vi "PublishCurrentValues.vi"(8 "error in (no error)":errorcluster, 10 "Qbus in":refnum<class "Qbus.lvclass">, 11 "config in":T1) -> (0 "error out":errorcluster, 3 "config out":T1)   [LabVIEW 2017, in "TestPanel.lvlib"]
uses:
  <vilib>/addons/InsightCM/Devices/Shared/Common/TestPanel/TestPanel.lvlib
  <vilib>/addons/InsightCM/Devices/Shared/Common/TestPanel/controls/Configuration.ctl
  <vilib>/addons/InsightCM/Devices/Shared/Common/TestPanel/controls/State.ctl
  <vilib>/addons/InsightCM/MessageBus/Base/controls/IRoutingSource.ctl
  <vilib>/addons/Qbus/Qbus.lvclass
  <vilib>/addons/InsightCM/MessageBus/MessageLibrary/Device/controls/DeviceTestPanelGetCurrentValuesResponseBody.ctl
  <vilib>/addons/InsightCM/MessageBus/Base/controls/TestPanelCurrentValues.ctl
  <vilib>/addons/InsightCM/MessageBus/Base/controls/KeyValuePair.ctl
  <vilib>/addons/InsightCM/MessageBus/Base/controls/TestPanelCurrentValue.ctl
  <vilib>/addons/InsightCM/MessageBus/Base/controls/TestPanelValue.ctl
  <vilib>/addons/InsightCM/Devices/Shared/Common/ServerComm/ServerComm.lvlib
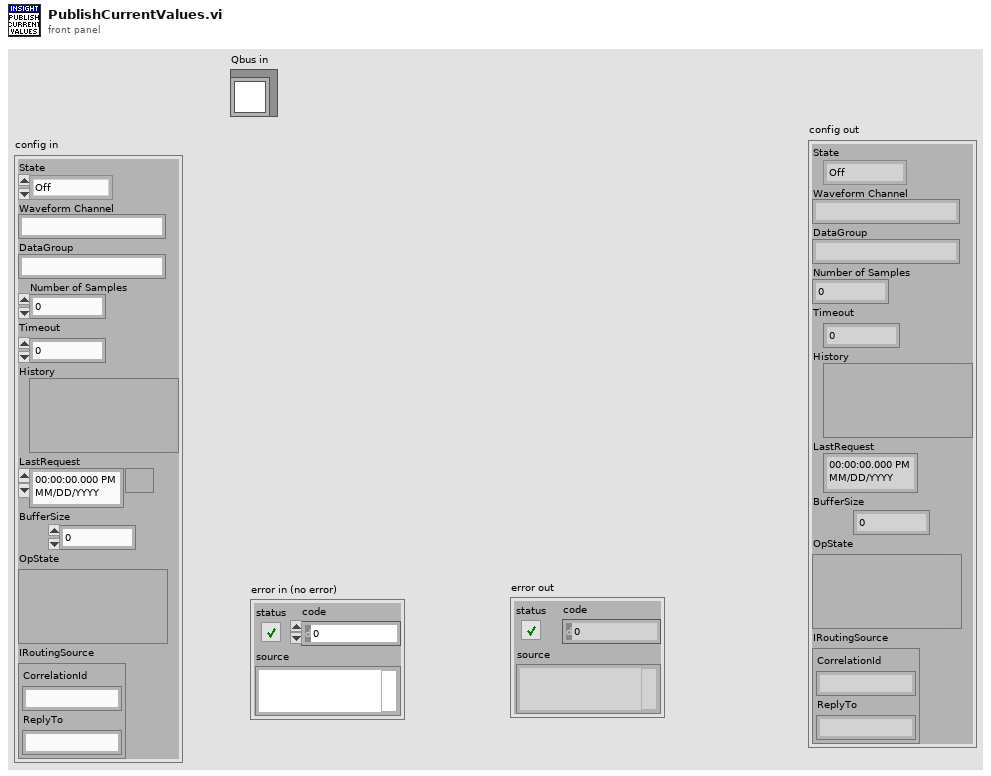
[diagram p1: front panel]
types:
  T1 = typedef "TestPanel.lvlib/Configuration.ctl" = cluster{"State":T2, "Waveform Channel":string, "DataGroup":string, "Number of Samples":i32, "Timeout":dbl, "History":variant, "LastRequest":timestamp, "BufferSize":i32, "OpState":variant, "IRoutingSource":T3}
  T2 = typedef "TestPanel.lvlib/State.ctl" = enum16{"Off", "On", "PendingValues", "PendingDataSet"}
  T3 = typedef "IRoutingSource.ctl" = cluster{"CorrelationId":string, "ReplyTo":string}
  T4 = typedef "DeviceTestPanelGetCurrentValuesResponseBody.ctl" = cluster{"Data":T5[]}
  T5 = typedef "TestPanelCurrentValues.ctl" = cluster{"DataGroup":string, "OperatingState":string, "ChannelStatus":T6[], "Values":T7[]}
  T6 = typedef "KeyValuePair.ctl" = cluster{"Key":string, "Value":string}
  T7 = typedef "TestPanelCurrentValue.ctl" = cluster{"TrendPointId":string, "AssetName":string, "MetricName":string, "Unit":string, "Value":T8}
  T8 = typedef "TestPanelValue.ctl" = cluster{"Value":dbl, "Timestamp":i64, "Invalid":bool}
  T9 = typedef "Message.ctl" = cluster{"Header":T10, "Body":u8[]}
  T10 = typedef "MessageHeader.ctl" = cluster{"MessageName":string, "Timestamp":i64, "CorrelationId":string, "ContentType":string, "RoutingKey":string, "Properties":T6[]}
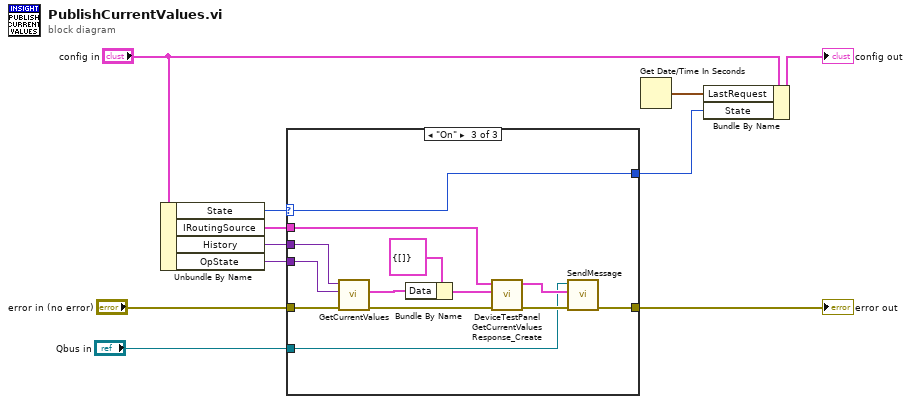
[diagram p0: block diagram]
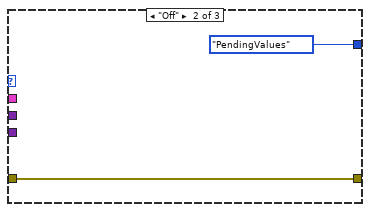
[diagram p3: hidden frame]
diagram:
  n1 = Unbundle By Name("config in") -> ("State"=w8:T2, "IRoutingSource"=w4:T3, "History"=w7:variant, "OpState"=w6:variant)
  n2 = case shown="\"On\"" w8 {
    selector: w8 -> [w13 _ w16]
    tunnel: w7 -> [_ _ w28]
    tunnel: w6 -> [_ _ w27]
    tunnel: "error in (no error)" -> [w12 w14 w23]
    tunnel: w4 -> [_ _ w21]
    tunnel: "Qbus in" -> [_ _ w18]
    tunnel: [w12 w14 w17] -> w2
    tunnel: [w13 State."PendingValues" ("State") w16] -> w1
    frame Default {
    }
    frame "Off" {
    }
    frame "On" {
      n3 = call <vilib>:"GetCurrentValues.vi"("error in (no error)"=w23, "OpState"=w27, "History"=w28) -> ("error out"=w22:errorcluster, "current values"=w25:T5[])  [unwired: 7 in]
      n4 = Bundle By Name(cluster=T4 {"Data"=[]} ("DeviceTestPanelGetCurrentValuesResponse"), "Data"=w25) -> (w24:T4)
      n5 = call <vilib>:"DeviceTestPanelGetCurrentValuesResponse_Create.vi"("error in (no error)"=w22, "DeviceTestPanelGetCurrentValuesResponse"=w24, "IRoutingSource"=w21) -> ("error out"=w20:errorcluster, "Message"=w19:T9)  [unwired: 7 in]
      n6 = call <vilib>:"SendMessage.vi"("error in (no error)"=w20, "message"=w19, "Qbus in"=w18) -> ("error out"=w17:errorcluster)  [unwired: 7 in, 1 out]
    }
  }
  "error out" <- w2
  n7 = Get Date/Time In Seconds() -> (seconds since 1Jan1904=w9:timestamp)
  n8 = Bundle By Name(cluster="config in", "LastRequest"=w9, "State"=w1) -> (→"config out":T1)
